vi "USB - Open Connection.vi"(8 "error in":errorcluster, 11 "COM Port":string) -> (0 "error out":errorcluster, 3 "VISA resource name out":refnum<visa-resource-name>)   [LabVIEW 2021]
uses:
  <vilib>/Instr/_visa.llb/VISA Configure Serial Port (Instr).vi
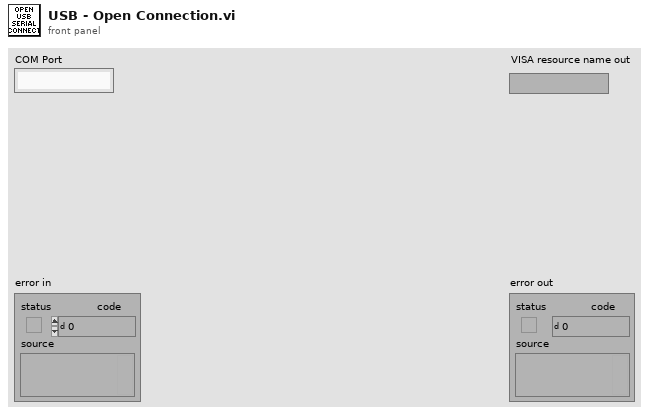
[diagram p1: front panel]
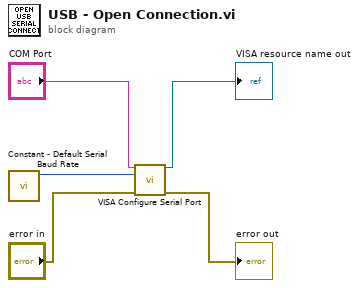
[diagram p0: block diagram]
diagram:
  n1 = call "Constant - Default Serial Baud Rate.vi"() -> ("Baud Rate"=w4:i32)  [unwired: 11 in]
  n2 = call-poly "VISA Configure Serial Port"("VISA resource name"="COM Port", "baud rate (9600)"=w4, "error in (no error)"="error in") -> ("VISA resource name out"=→"VISA resource name out":refnum<visa-resource-name>, "error out"=→"error out":errorcluster)  [unwired: 11 in]
